vi "Database Update Value.vi"(6 "data":variant, 7 "condition":string, 8 "error in (no error)":errorcluster, 9 "columns":string[](array[string]), 10 "table":string, 11 "Database in":refnum<class "DatabaseAPI.lvclass">) -> (0 "error out":errorcluster, 3 "Database out":refnum<class "DatabaseAPI.lvclass">)   [LabVIEW 2015, in "DatabaseAPI.lvclass"]
uses:
  DatabaseAPI.lvclass
  DatabaseAPI.lvclass/DatabaseAPI.ctl
  <vilib>/addons/database/Connection.llb/DB Tools Open Connec (String).vi
  <vilib>/addons/database/NI_Database_API.lvlib
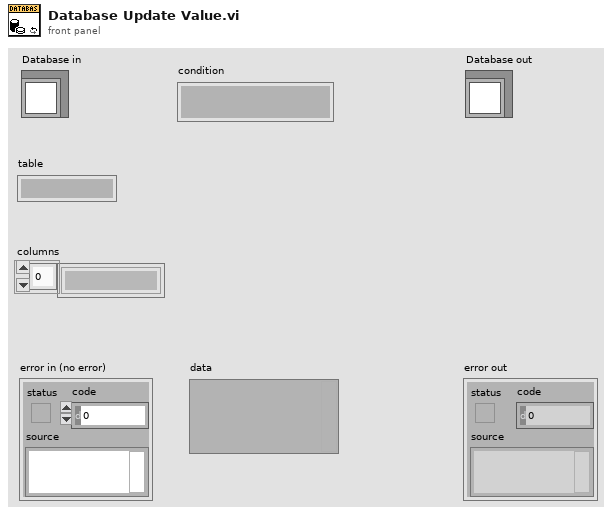
[diagram p1: front panel]
types:
  T1 = typedef "NI_Database_API.lvlib/Conn ObjectReference.ctl" = refnum<k1>
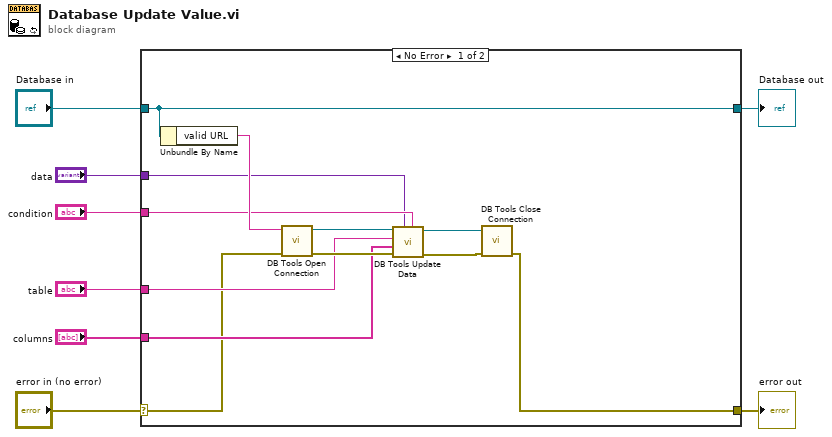
[diagram p0: block diagram]
diagram:
  n1 = case shown="No Error" "error in (no error)" {
    selector: "error in (no error)" -> [w10 w22]
    tunnel: [w9 w22] -> w7
    tunnel: [w20 w21] -> w5
    tunnel: "Database in" -> [w20 w21]
    tunnel: "table" -> [w16 _]
    tunnel: "condition" -> [w15 _]
    tunnel: "data" -> [w14 _]
    tunnel: "columns" -> [w13 _]
    frame No Error {
      n2 = Unbundle By Name(w20) -> ("valid URL"=w19:string)
      n3 = call-poly <vilib>:"DB Tools Open Connection.vi"("error in (no error)"=w10, "connection information"=w19) -> ("error out"=w17:errorcluster, "connection reference"=w18:T1)  [unwired: 6 in]
      n4 = call <vilib>:"DB Tools Update Data.vi"("condition"=w15, "data"=w14, "error in (no error)"=w17, "columns"=w13, "table"=w16, "connection reference"=w18) -> ("error out"=w11:errorcluster, "connection reference out"=w12:T1)  [unwired: 4 in]
      n5 = call <vilib>:"DB Tools Close Connection.vi"("error in (no error)"=w11, "connection reference"=w12) -> ("error out"=w9:errorcluster)  [unwired: 5 in]
    }
    frame Error {
    }
  }
  "error out" <- w7
  "Database out" <- w5
